vi "ReadCfg.vi"() -> (14 "data":T1)   [LabVIEW 2018]
uses:
  ControlCfg.ctl
  ControlConfigMisura.ctl
  ControlConfigDI.ctl
  <vilib>/Utility/config.llb/NI_LVConfig.lvlib
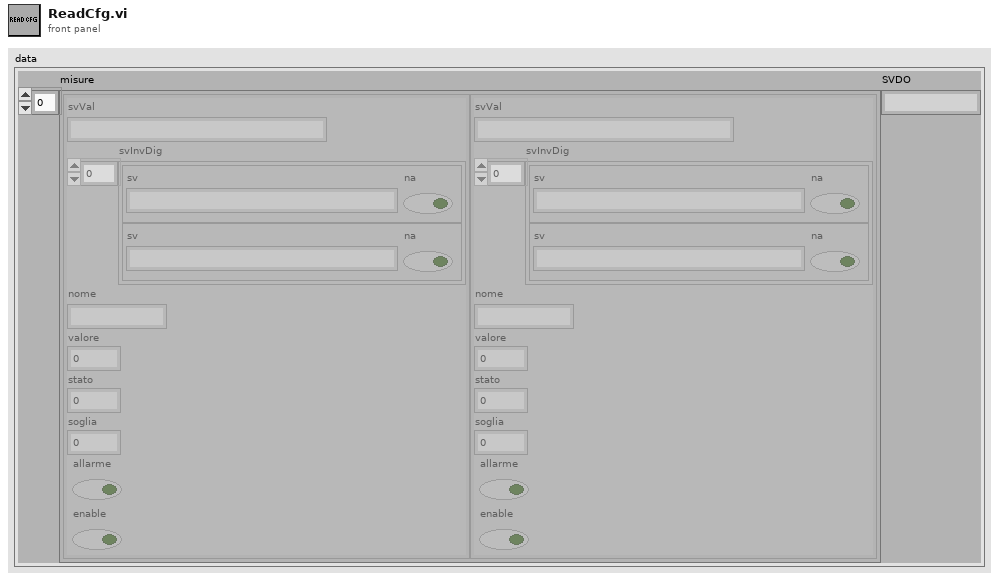
[diagram p1: front panel]
types:
  T1 = typedef "ControlCfg.ctl" = cluster{"misure":T2[], "SVDO":string}
  T2 = typedef "ControlConfigMisura.ctl" = cluster{"svVal":string, "svInvDig":T3[], "nome":string, "valore":dbl, "stato":i16, "soglia":dbl, "allarme":bool, "enable":bool}
  T3 = typedef "ControlConfigDI.ctl" = cluster{"sv":string, "na":bool}
  T4 = typedef "NI_LVConfig.lvlib/Config Data RefNum.ctl" = refnum<k1>
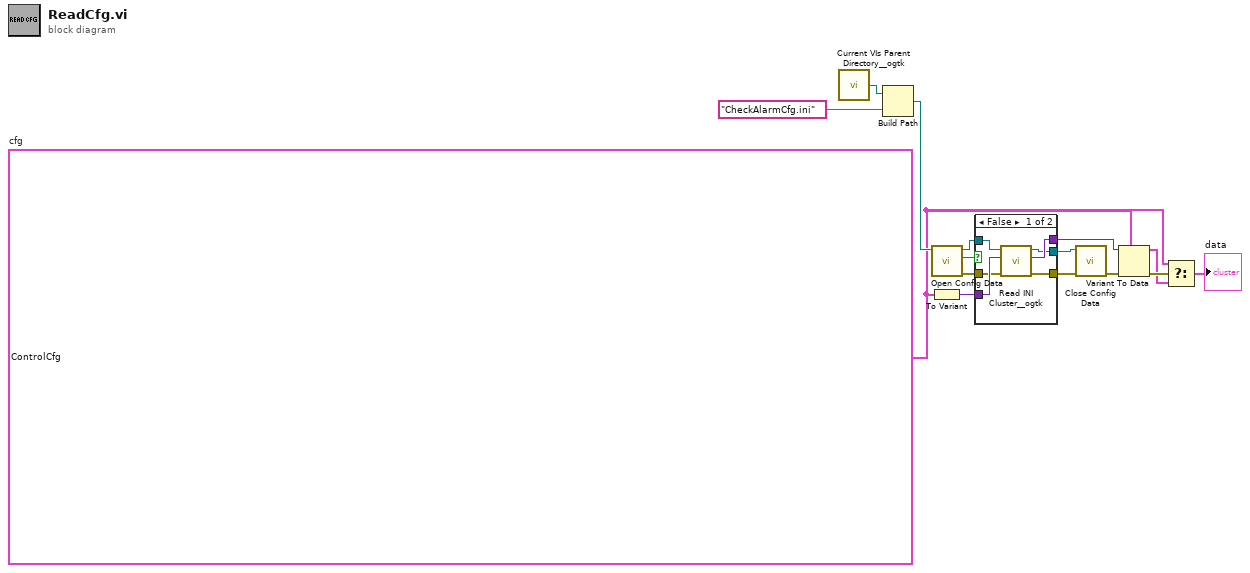
[diagram p0: block diagram]
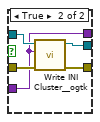
[diagram p2: hidden frame]
diagram:
  w3 = T1 {"misure"=[{"svVal"="\\\\localhost\\Sample\\p14", "svInvDig"=[{"sv"="\\\\localhost\\ADAM5000_DI_S3\\DI_07", "na"=FALSE}, {"sv"="\\\\localhost\\ADAM5000_DI_S2\\DI_04", "na"=TRUE}, {"sv"="\\\\localhost\\ADAM5000_DI_S2\\DI_05", "na"=TRUE}, {"sv"="\\\\localhost\\ADAM5000_DI_S2\\DI_00", "na"=TRUE}], "nome"="Polveri 14", "valore"=0.0, "stato"=0, "soglia"=4.0, "allarme"=FALSE, "enable"=TRUE}, {"svVal"="\\\\localhost\\Sample\\p18", "svInvDig"=[{"sv"="\\\\localhost\\ADAM5000_DI_S3\\DI_09", "na"=FALSE}, {"sv"="\\\\localhost\\ADAM5000_DI_S2\\DI_02", "na"=TRUE}, {"sv"="\\\\localhost\\ADAM5000_DI_S2\\DI_03", "na"=TRUE}, {"sv"="\\\\localhost\\ADAM5000_DI_S2\\DI_00", "na"=TRUE}], "nome"="Polveri 18", "valore"=0.0, "stato"=0, "soglia"=4.0, "allarme"=FALSE, "enable"=TRUE}, {"svVal"="\\\\localhost\\Sample\\p16", "svInvDig"=[{"sv"="\\\\localhost\\ADAM5000_DI_S2\\DI_13", "na"=TRUE}, {"sv"="\\\\localhost\\ADAM5000_DI_S2\\DI_14", "na"=TRUE}, {"sv"="\\\\localhost\\StatiModbus\\stsADAM", "na"=FALSE}, {"sv"="\\\\localhost\\ADAM5000_DI_S3\\DI_05", "na"=FALSE}], "nome"="Polveri 16", "valore"=0.0, "stato"=0, "soglia"=4.0, "allarme"=FALSE, "enable"=TRUE}, {"svVal"="\\\\localhost\\Sample\\so2", "svInvDig"=[{"sv"="\\\\localhost\\ADAM5000_DI_S3\\DI_05", "na"=FALSE}, {"sv"="\\\\localhost\\FTIR\\Allarme", "na"=FALSE}, {"sv"="\\\\localhost\\FTIR\\Zero", "na"=FALSE}, {"sv"="\\\\localhost\\FTIR\\Maintenance", "na"=FALSE}, {"sv"="\\\\localhost\\ADAM5000_DI_S2\\DI_01", "na"=FALSE}, {"sv"="\\\\localhost\\ADAM5000_DI_S2\\DI_07", "na"=FALSE}, {"sv"="\\\\localhost\\ADAM5000_DI_S2\\DI_08", "na"=FALSE}, {"sv"="\\\\localhost\\ADAM5000_DI_S2\\DI_09", "na"=FALSE}, {"sv"="\\\\localhost\\ADAM5000_DO_S4\\DO_00", "na"=TRUE}], "nome"="SO2", "valore"=0.0, "stato"=0, "soglia"=160.0, "allarme"=FALSE, "enable"=TRUE}, {"svVal"="\\\\localhost\\Sample\\nox", "svInvDig"=[{"sv"="\\\\localhost\\ADAM5000_DI_S3\\DI_05", "na"=FALSE}, {"sv"="\\\\localhost\\FTIR\\Allarme", "na"=FALSE}, {"sv"="\\\\localhost\\FTIR\\Zero", "na"=FALSE}, {"sv"="\\\\localhost\\FTIR\\Maintenance", "na"=FALSE}, {"sv"="\\\\localhost\\ADAM5000_DI_S2\\DI_01", "na"=FALSE}, {"sv"="\\\\localhost\\ADAM5000_DI_S2\\DI_07", "na"=FALSE}, {"sv"="\\\\localhost\\ADAM5000_DI_S2\\DI_08", "na"=FALSE}, {"sv"="\\\\localhost\\ADAM5000_DI_S2\\DI_09", "na"=FALSE}, {"sv"="\\\\localhost\\ADAM5000_DO_S4\\DO_00", "na"=TRUE}], "nome"="NOX", "valore"=0.0, "stato"=0, "soglia"=280.0, "allarme"=FALSE, "enable"=TRUE}, {"svVal"="\\\\localhost\\Sample\\cot", "svInvDig"=[{"sv"="\\\\localhost\\ADAM5000_DI_S3\\DI_05", "na"=FALSE}, {"sv"="\\\\localhost\\ADAM5000_DI_S2\\DI_01", "na"=FALSE}, {"sv"="\\\\localhost\\ADAM5000_DI_S2\\DI_07", "na"=FALSE}, {"sv"="\\\\localhost\\ADAM5000_DI_S2\\DI_08", "na"=FALSE}, {"sv"="\\\\localhost\\ADAM5000_DI_S2\\DI_09", "na"=FALSE}, {"sv"="\\\\localhost\\ADAM5000_DI_S2\\DI_09", "na"=TRUE}, {"sv"="\\\\localhost\\ADAM5000_DO_S4\\DO_00", "na"=TRUE}], "nome"="COT", "valore"=0.0, "stato"=0, "soglia"=16.0, "allarme"=FALSE, "enable"=TRUE}, {"svVal"="\\\\localhost\\Sample\\hcl", "svInvDig"=[{"sv"="\\\\localhost\\ADAM5000_DI_S3\\DI_05", "na"=FALSE}, {"sv"="\\\\localhost\\FTIR\\Allarme", "na"=FALSE}, {"sv"="\\\\localhost\\FTIR\\Zero", "na"=FALSE}, {"sv"="\\\\localhost\\FTIR\\Maintenance", "na"=FALSE}, {"sv"="\\\\localhost\\ADAM5000_DI_S2\\DI_01", "na"=FALSE}, {"sv"="\\\\localhost\\ADAM5000_DI_S2\\DI_07", "na"=FALSE}, {"sv"="\\\\localhost\\ADAM5000_DI_S2\\DI_08", "na"=FALSE}, {"sv"="\\\\localhost\\ADAM5000_DI_S2\\DI_09", "na"=FALSE}, {"sv"="\\\\localhost\\ADAM5000_DO_S4\\DO_00", "na"=TRUE}], "nome"="HCL", "valore"=0.0, "stato"=0, "soglia"=40.0, "allarme"=FALSE, "enable"=TRUE}, {"svVal"="\\\\localhost\\Sample\\hf", "svInvDig"=[{"sv"="\\\\localhost\\ADAM5000_DI_S3\\DI_05", "na"=FALSE}, {"sv"="\\\\localhost\\FTIR\\Allarme", "na"=FALSE}, {"sv"="\\\\localhost\\FTIR\\Zero", "na"=FALSE}, {"sv"="\\\\localhost\\FTIR\\Maintenance", "na"=FALSE}, {"sv"="\\\\localhost\\ADAM5000_DI_S2\\DI_01", "na"=FALSE}, {"sv"="\\\\localhost\\ADAM5000_DI_S2\\DI_07", "na"=FALSE}, {"sv"="\\\\localhost\\ADAM5000_DI_S2\\DI_08", "na"=FALSE}, {"sv"="\\\\localhost\\ADAM5000_DI_S2\\DI_09", "na"=FALSE}, {"sv"="\\\\localhost\\ADAM5000_DO_S4\\DO_00", "na"=TRUE}], "nome"="HF", "valore"=0.0, "stato"=0, "soglia"=1.6, "allarme"=FALSE, "enable"=FALSE}], "SVDO"="\\\\localhost\\Sample\\AlarmDO"}  # cfg
  n1 = call <userlib>:"Current VIs Parent Directory__ogtk.vi"() -> ("Parent Directory (+ Relative)"=w7:path)  [unwired: 5 in]
  n2 = Build Path(base path=w7, name or relative path="CheckAlarmCfg.ini") -> (appended path=w5:path)
  n3 = call <vilib>:"Open Config Data.vi"("configuration file path"=w5) -> ("error out"=w13:errorcluster, "file created?"=w15:bool, "refnum"=w12:T4)  [unwired: 8 in]
  n4 = To Variant(anything=w3) -> (Variant=w14:variant)
  n5 = case shown="False" w15 {
    tunnel: w14 -> [w20 w22]
    tunnel: w13 -> [w17 w26]
    tunnel: w12 -> [w21 w25]
    tunnel: [w18 w24] -> w11
    tunnel: [w16 w23] -> w10
    tunnel: [w19 w22] -> w9
    frame False {
      n6 = call <userlib>:"Read INI Cluster__ogtk.vi"("error in (no error)"=w17, "INI Fomatted Cluster Type"=w20, "refnum"=w21) -> ("error out"=w16:errorcluster, "INI Fomatted Cluster"=w19:variant, "dup refnum"=w18:T4)  [unwired: 4 in, 2 out]
    }
    frame True {
      n7 = call <userlib>:"Write INI Cluster__ogtk.vi"("error in (no error)"=w26, "INI Fomatted Cluster"=w22, "refnum"=w25) -> ("error out"=w23:errorcluster, "dup refnum"=w24:T4)  [unwired: 7 in]
    }
  }
  n8 = call <vilib>:"Close Config Data.vi"("error in (no error)"=w10, "refnum"=w11) -> ("error out"=w8:errorcluster)  [unwired: 8 in, 1 out]
  n9 = Variant To Data(error in=w8, type=w3, Variant=w9) -> (data=w2:T1, error out=w4:errorcluster)
  n10 = Select(t=w3, s=w4, f=w2) -> (s? t:f=→"data":T1)
